vi "Slave_T.vi"() -> ()   [LabVIEW 2017, in "Konfiguracja.lvlib"]
uses:
  Libraries/Konfiguracja/Konfiguracja.lvlib
  Controls/Enum_SM_read_input_write.ctl
  <vilib>/Utility/config.llb/NI_LVConfig.lvlib
panel:
  in  "System Tab":enum32{"Termometry"}(tab)
  in  "Etykiety T1-10":T1
  in  "Moduł aktywny":bool
  in  "Identyfikator slave'a":dbl=2.0 min=2.0 max=127.0 step=1.0
  in  "Copy":bool
  in  "Save":bool
  in  "T10O":dbl
  in  "T10A":dbl
  in  "T9O":dbl
  in  "T9A":dbl
  in  "T8O":dbl
  in  "T8A":dbl
  in  "T7O":dbl
  in  "T7A":dbl
  in  "T6O":dbl
  in  "T6A":dbl
  in  "T5O":dbl
  in  "T5A":dbl
  in  "T4O":dbl
  in  "T4A":dbl
  in  "T3O":dbl
  in  "T3A":dbl
  in  "T2O":dbl
  in  "T2A":dbl
  in  "T1O":dbl
  in  "T1A":dbl
  in  "Termometr 10":bool
  in  "Termometr 9":bool
  in  "Termometr 8":bool
  in  "Termometr 7":bool
  in  "Termometr 6":bool caption="Termometr 1"
  in  "Termometr 5":bool
  in  "Termometr 4":bool
  in  "Termometr 3":bool
  in  "Termometr 2":bool
  in  "Termometr 1":bool
  # "Etykieta"
  # "Kopiuje wartośc zadaną z \npola 1 do pozostałych"
  # "Zadana wartość\nostrzegawcza"
  # "Zadana wartość \nalarmowa"
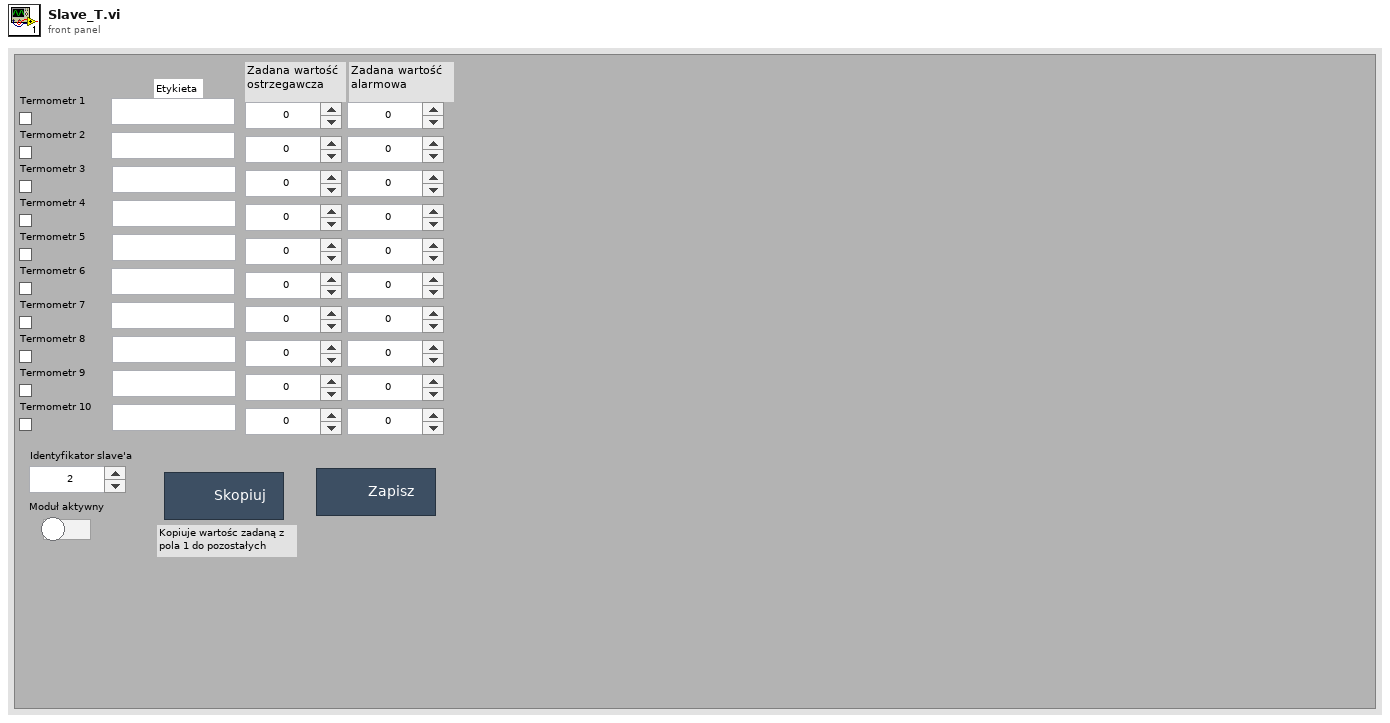
[diagram p1: front panel]
types:
  T1 = cluster{"Termometr 1":string, "Termometr 2":string, "Termometr 3":string, "Termometr 4":string, "Termometr 5":string, "Termometr 6":string, "Termometr 7":string, "Termometr 8":string, "Termometr 9":string, "Termometr 10":string}
  T2 = typedef "Konfiguracja.lvlib/Enum_SM_read_input_write.ctl" = enum16{"Load", "Wait for input", "Input", "Copy", "Write", "Exit"}
  T3 = typedef "Konfiguracja.lvlib/Tx.ctl" = cluster{"Termometr 1":bool, "Termometr 2":bool, "Termometr 3":bool, "Termometr 4":bool, "Termometr 5":bool, "Termometr 6":bool, "Termometr 7":bool, "Termometr 8":bool, "Termometr 9":bool, "Termometr 10":bool, "Termometr 11":bool, "Termometr 12":bool, "Termometr 13":bool, "Termometr 14":bool, "Termometr 15":bool, "Termometr 16":bool, "Termometr 17":bool, "Termometr 18":bool, "Termometr 19":bool, "Termometr 20":bool}
  T4 = typedef "Konfiguracja.lvlib/TxO.ctl" = cluster{"T1O":dbl, "T2O":dbl, "T3O":dbl, "T4O":dbl, "T5O":dbl, "T6O":dbl, "T7O":dbl, "T8O":dbl, "T9O":dbl, "T10O":dbl, "T11O":dbl, "T12O":dbl, "T13O":dbl, "T14O":dbl, "T15O":dbl, "T16O":dbl, "T17O":dbl, "T18O":dbl, "T19O":dbl, "T20O":dbl}
  T5 = typedef "Konfiguracja.lvlib/TxA.ctl" = cluster{"T1A":dbl, "T2A":dbl, "T3A":dbl, "T4A":dbl, "T5A":dbl, "T6A":dbl, "T7A":dbl, "T8A":dbl, "T9A":dbl, "T10A":dbl, "T11A":dbl, "T12A":dbl, "T13A":dbl, "T14A":dbl, "T15A":dbl, "T16A":dbl, "T17A":dbl, "T18A":dbl, "T19A":dbl, "T20A":dbl}
  T6 = cluster{"Termometr 1":bool, "Termometr 2":bool, "Termometr 3":bool, "Termometr 4":bool, "Termometr 5":bool, "Termometr 6":bool, "Termometr 7":bool, "Termometr 8":bool, "Termometr 9":bool, "Termometr 10":bool}
  T7 = cluster{"T1O":dbl, "T2O":dbl, "T3O":dbl, "T4O":dbl, "T5O":dbl, "T6O":dbl, "T7O":dbl, "T8O":dbl, "T9O":dbl, "T10O":dbl}
  T8 = cluster{"T1A":dbl, "T2A":dbl, "T3A":dbl, "T4A":dbl, "T5A":dbl, "T6A":dbl, "T7A":dbl, "T8A":dbl, "T9A":dbl, "T10A":dbl}
  T9 = cluster{cluster{"T1A":dbl, "T2A":dbl, "T3A":dbl, "T4A":dbl, "T5A":dbl, "T6A":dbl, "T7A":dbl, "T8A":dbl, "T9A":dbl, "T10A":dbl}, cluster{"T1O":dbl, "T2O":dbl, "T3O":dbl, "T4O":dbl, "T5O":dbl, "T6O":dbl, "T7O":dbl, "T8O":dbl, "T9O":dbl, "T10O":dbl}, cluster{"Termometr 1":bool, "Termometr 2":bool, "Termometr 3":bool, "Termometr 4":bool, "Termometr 5":bool, "Termometr 6":bool, "Termometr 7":bool, "Termometr 8":bool, "Termometr 9":bool, "Termometr 10":bool}, "Moduł aktywny":bool, "Etykiety T1-10":cluster{"Termometr 1":string, "Termometr 2":string, "Termometr 3":string, "Termometr 4":string, "Termometr 5":string, "Termometr 6":string, "Termometr 7":string, "Termometr 8":string, "Termometr 9":string, "Termometr 10":string}}
  T10 = typedef "NI_LVConfig.lvlib/Config Data RefNum.ctl" = refnum<k1>
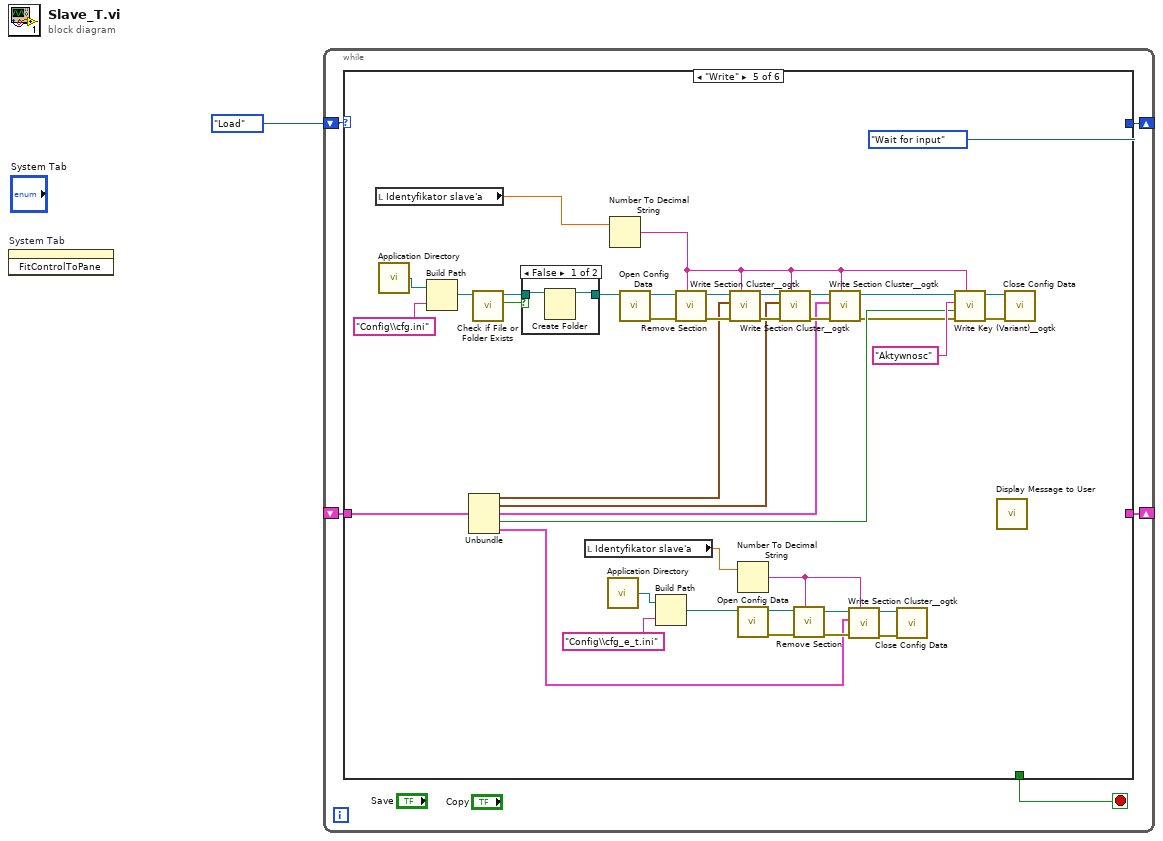
[diagram p0: block diagram]
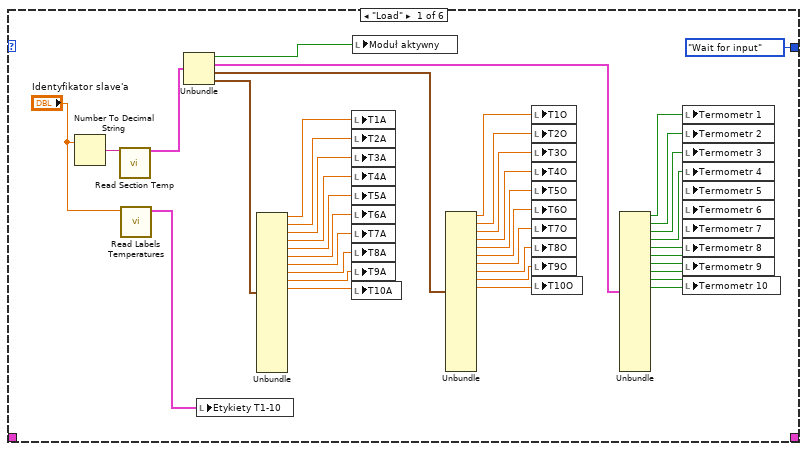
[diagram p2: hidden frame]
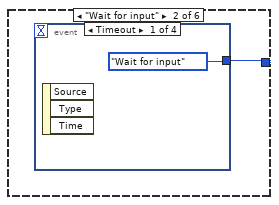
[diagram p3: hidden frame]
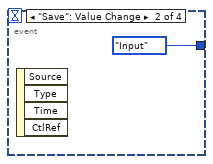
[diagram p4: hidden frame]
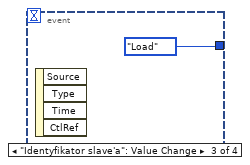
[diagram p5: hidden frame]
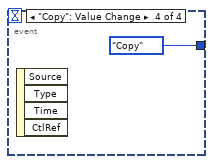
[diagram p6: hidden frame]
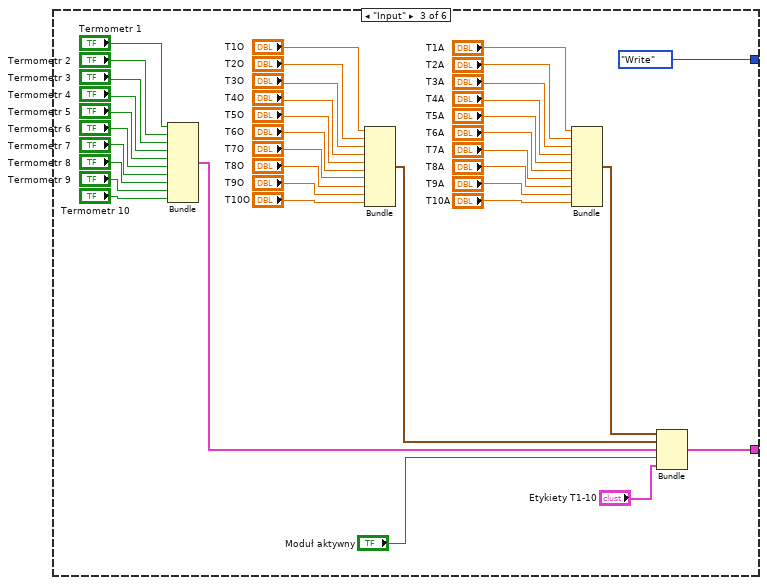
[diagram p7: hidden frame]
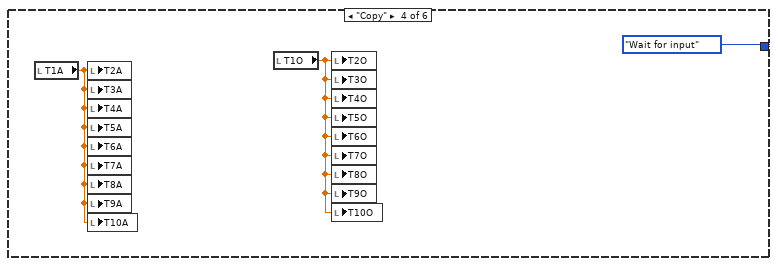
[diagram p8: hidden frame]
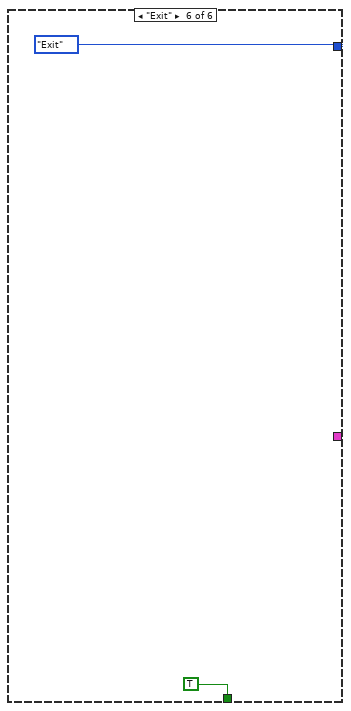
[diagram p10: hidden frame]
diagram:
  n1 = invoke on="System Tab" class="TabCtl (strict)" method="FitControlToPane"() -> ()  [unwired: 3 in, 3 out]
  n2 = while {
    shift-right: [w5] -> _
    shift-left: Enum_SM_read_input_write."Load" -> [w6]
    shift-right: [w4] -> _
    shift-left: _ -> [w3]
    stop <- w2 stop-if-true
    n3 = case shown="\"Write\"" w6 {
      tunnel: [Enum_SM_read_input_write."Wait for input" w46 Enum_SM_read_input_write."Write" Enum_SM_read_input_write."Wait for input" Enum_SM_read_input_write."Wait for input" Enum_SM_read_input_write."Exit"] -> w5
      tunnel: [_ _ w54 _ _ _] -> w4
      tunnel: w3 -> [_ _ _ _ w126 _]
      tunnel: [_ _ _ _ _ TRUE] -> w2
      frame "Load" {
        n4 = Number To Decimal String(number="Identyfikator slave'a") -> (decimal integer string=w13:string)  [unwired: 1 in]
        n5 = call "Read Section Temp.vi"("section"=w13) -> ("Data Cluster"=w14:cluster{bool, "Tx":T3, "TxO":T4, "TxA":T5})  [unwired: 14 in]
        n6 = call "Read Labels Temperatures.vi"("Slave ID"="Identyfikator slave'a") -> ("Etykiety T1-10"=w7:T1)  [unwired: 10 in]
        n7 = Unbundle(w14) -> (w9:bool, "Tx"=w10:T3, "TxO"=w11:T4, "TxA"=w12:T5)
        n8 = local write "Etykiety T1-10"(w7) -> ()
        n9 = Unbundle(w12) -> ("T1A"=w36:dbl, "T2A"=w37:dbl, "T3A"=w38:dbl, "T4A"=w39:dbl, "T5A"=w40:dbl, "T6A"=w41:dbl, "T7A"=w42:dbl, "T8A"=w43:dbl, "T9A"=w44:dbl, "T10A"=w45:dbl)  [unwired: 10 out]
        n10 = local write "T1A"(w36) -> ()
        n11 = local write "T2A"(w37) -> ()
        n12 = local write "T3A"(w38) -> ()
        n13 = local write "T4A"(w39) -> ()
        n14 = local write "T5A"(w40) -> ()
        n15 = local write "T6A"(w41) -> ()
        n16 = local write "T7A"(w42) -> ()
        n17 = local write "T8A"(w43) -> ()
        n18 = local write "T9A"(w44) -> ()
        n19 = local write "T10A"(w45) -> ()
        n20 = local write "Moduł aktywny"(w9) -> ()
        n21 = Unbundle(w11) -> ("T1O"=w26:dbl, "T2O"=w27:dbl, "T3O"=w28:dbl, "T4O"=w29:dbl, "T5O"=w30:dbl, "T6O"=w31:dbl, "T7O"=w32:dbl, "T8O"=w33:dbl, "T9O"=w34:dbl, "T10O"=w35:dbl)  [unwired: 10 out]
        n22 = local write "T1O"(w26) -> ()
        n23 = local write "T2O"(w27) -> ()
        n24 = local write "T3O"(w28) -> ()
        n25 = local write "T4O"(w29) -> ()
        n26 = local write "T5O"(w30) -> ()
        n27 = local write "T6O"(w31) -> ()
        n28 = local write "T7O"(w32) -> ()
        n29 = local write "T8O"(w33) -> ()
        n30 = local write "T9O"(w34) -> ()
        n31 = local write "T10O"(w35) -> ()
        n32 = Unbundle(w10) -> ("Termometr 1"=w16:bool, "Termometr 2"=w17:bool, "Termometr 3"=w18:bool, "Termometr 4"=w19:bool, "Termometr 5"=w20:bool, "Termometr 6"=w21:bool, "Termometr 7"=w22:bool, "Termometr 8"=w23:bool, "Termometr 9"=w24:bool, "Termometr 10"=w25:bool)  [unwired: 10 out]
        n33 = local write "Termometr 1"(w16) -> ()
        n34 = local write "Termometr 2"(w17) -> ()
        n35 = local write "Termometr 3"(w18) -> ()
        n36 = local write "Termometr 4"(w19) -> ()
        n37 = local write "Termometr 5"(w20) -> ()
        n38 = local write "Termometr 6"(w21) -> ()
        n39 = local write "Termometr 7"(w22) -> ()
        n40 = local write "Termometr 8"(w23) -> ()
        n41 = local write "Termometr 9"(w24) -> ()
        n42 = local write "Termometr 10"(w25) -> ()
      }
      frame "Wait for input" {
        n43 = event shown="[0] Timeout" {
          selector: _ -> [_ _ _ _]
          dyn-events: _ -> [_ _ _ _]
          timeout: _ -> [_ _ _ _]
          tunnel: [Enum_SM_read_input_write."Wait for input" Enum_SM_read_input_write."Input" Enum_SM_read_input_write."Load" Enum_SM_read_input_write."Copy"] -> w46
          event Timeout {
            n44 = event-data() -> ()  [unwired: 1 in, 3 out]
          }
          event "Save": Value Change {
            n45 = event-data() -> ()  [unwired: 1 in, 4 out]
          }
          event "Identyfikator slave'a": Value Change {
            n46 = event-data() -> ()  [unwired: 1 in, 4 out]
          }
          event "Copy": Value Change {
            n47 = event-data() -> ()  [unwired: 1 in, 4 out]
          }
        }
      }
      frame "Input" {
        n48 = Bundle("Termometr 1"="Termometr 1", "Termometr 2"="Termometr 2", "Termometr 3"="Termometr 3", "Termometr 4"="Termometr 4", "Termometr 5"="Termometr 5", "Termometr 6"="Termometr 6", "Termometr 7"="Termometr 7", "Termometr 8"="Termometr 8", "Termometr 9"="Termometr 9", "Termometr 10"="Termometr 10") -> (w55:T6)  [unwired: 1 in]
        n49 = Bundle("T1O"="T1O", "T2O"="T2O", "T3O"="T3O", "T4O"="T4O", "T5O"="T5O", "T6O"="T6O", "T7O"="T7O", "T8O"="T8O", "T9O"="T9O", "T10O"="T10O") -> (w56:T7)  [unwired: 1 in]
        n50 = Bundle("T1A"="T1A", "T2A"="T2A", "T3A"="T3A", "T4A"="T4A", "T5A"="T5A", "T6A"="T6A", "T7A"="T7A", "T8A"="T8A", "T9A"="T9A", "T10A"="T10A") -> (w57:T8)  [unwired: 1 in]
        n51 = Bundle(w57, w56, w55, "Moduł aktywny"="Moduł aktywny", "Etykiety T1-10"="Etykiety T1-10") -> (w54:T9)  [unwired: 1 in]
      }
      frame "Copy" {
        n52 = local read "T1A"() -> (w89:dbl)
        n53 = local write "T2A"(w89) -> ()
        n54 = local write "T3A"(w89) -> ()
        n55 = local write "T4A"(w89) -> ()
        n56 = local write "T5A"(w89) -> ()
        n57 = local write "T6A"(w89) -> ()
        n58 = local write "T7A"(w89) -> ()
        n59 = local write "T8A"(w89) -> ()
        n60 = local write "T9A"(w89) -> ()
        n61 = local write "T10A"(w89) -> ()
        n62 = local read "T1O"() -> (w88:dbl)
        n63 = local write "T2O"(w88) -> ()
        n64 = local write "T3O"(w88) -> ()
        n65 = local write "T4O"(w88) -> ()
        n66 = local write "T5O"(w88) -> ()
        n67 = local write "T6O"(w88) -> ()
        n68 = local write "T7O"(w88) -> ()
        n69 = local write "T8O"(w88) -> ()
        n70 = local write "T9O"(w88) -> ()
        n71 = local write "T10O"(w88) -> ()
      }
      frame "Write" {
        n72 = local read "Identyfikator slave'a"() -> (w114:dbl)
        n73 = call <vilib>:"Application Directory.vi"() -> ("Application Directory"=w128:path)
        n74 = Build Path(base path=w128, name or relative path="Config\\cfg.ini") -> (appended path=w91:path)
        n75 = Unbundle(w126) -> (w117:T8, w116:T7, w115:T6, "Moduł aktywny"=w111:bool, "Etykiety T1-10"=w95:T1)
        n76 = call <vilib>:"Check if File or Folder Exists.vi"("path"=w91) -> ("file or folder exists?"=w94:bool, "dup path"=w93:path)  [unwired: 8 in, 1 out]
        n77 = case shown="False" w94 {
          tunnel: w93 -> [w131 w132]
          tunnel: [w130 w132] -> w92
          frame False {
            n78 = Create Folder(path (use dialog)=w131) -> (created path=w130:path)  [unwired: 2 in, 2 out]
          }
          frame True {
          }
        }
        n79 = local read "Identyfikator slave'a"() -> (w101:dbl)
        n80 = call <vilib>:"Application Directory.vi"() -> ("Application Directory"=w102:path)
        n81 = Number To Decimal String(number=w114) -> (decimal integer string=w112:string)  [unwired: 1 in]
        n82 = call <vilib>:"Open Config Data.vi"("configuration file path"=w92) -> ("error out"=w118:errorcluster, "refnum"=w121:T10)  [unwired: 8 in, 1 out]
        n83 = Build Path(base path=w102, name or relative path="Config\\cfg_e_t.ini") -> (appended path=w105:path)
        n84 = call <vilib>:"Remove Section.vi"("section"=w112, "error in (no error)"=w118, "refnum"=w121) -> ("error out"=w119:errorcluster, "refnum out"=w120:T10)  [unwired: 6 in, 1 out]
        n85 = call <userlib>:"Write Section Cluster__ogtk.vi"("section (optional)"=w112, "error in (no error)"=w119, "Section Formatted Cluster"=w117, "refnum"=w120) -> ("error out"=w123:errorcluster, "dup refnum"=w125:T10)  [unwired: 6 in]
        n86 = Number To Decimal String(number=w101) -> (decimal integer string=w100:string)  [unwired: 1 in]
        n87 = call <vilib>:"Open Config Data.vi"("configuration file path"=w105) -> ("error out"=w103:errorcluster, "refnum"=w104:T10)  [unwired: 8 in, 1 out]
        n88 = call <userlib>:"Write Section Cluster__ogtk.vi"("section (optional)"=w112, "error in (no error)"=w123, "Section Formatted Cluster"=w116, "refnum"=w125) -> ("error out"=w122:errorcluster, "dup refnum"=w124:T10)  [unwired: 6 in]
        n89 = call <vilib>:"Remove Section.vi"("section"=w100, "error in (no error)"=w103, "refnum"=w104) -> ("error out"=w98:errorcluster, "refnum out"=w99:T10)  [unwired: 6 in, 1 out]
        n90 = call <userlib>:"Write Section Cluster__ogtk.vi"("section (optional)"=w112, "error in (no error)"=w122, "Section Formatted Cluster"=w115, "refnum"=w124) -> ("error out"=w110:errorcluster, "dup refnum"=w109:T10)  [unwired: 6 in]
        n91 = call <userlib>:"Write Section Cluster__ogtk.vi"("section (optional)"=w100, "error in (no error)"=w98, "Section Formatted Cluster"=w95, "refnum"=w99) -> ("error out"=w97:errorcluster, "dup refnum"=w96:T10)  [unwired: 6 in]
        n92 = call <vilib>:"Close Config Data.vi"("error in (no error)"=w97, "refnum"=w96) -> ()  [unwired: 8 in, 2 out]
        n93 = call <userlib>:"Write Key (Variant)__ogtk.vi"("section"=w112, "error in (no error)"=w110, "key-value"=w111, "key (optional)"="Aktywnosc", "refnum"=w109) -> ("error out"=w107:errorcluster, "refnum out"=w108:T10)  [unwired: 5 in]
        n94 = call "Display Message to User"() -> ()  [unwired: 10 in, 2 out]
        n95 = call <vilib>:"Close Config Data.vi"("error in (no error)"=w107, "refnum"=w108) -> ()  [unwired: 8 in, 2 out]
      }
      frame "Exit" {
      }
    }
  }
